vi "Gaussian surface parameter estimate.vi"(7 "output cluster":T1, 10 "X":dbl[](array[numeric]), 11 "Y":dbl[](array[numeric])) -> (3 "estimated parameters":dbl[](array[numeric]))   [LabVIEW 2023]
doc: "Estimate Gaussian surface parameters."
uses:
  <vilib>/Native 3D Graph/xcontrol/3DPC_SurfacePlot.xctl
  <vilib>/Analysis/NI_AALPro.lvlib
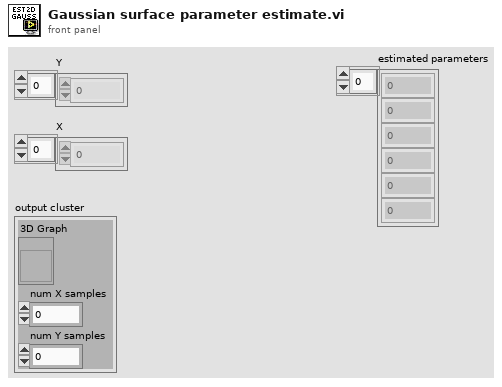
[diagram p1: front panel]
types:
  T1 = cluster{"3D Graph":refnum<vi>, "num X samples":i32, "num Y samples":i32}
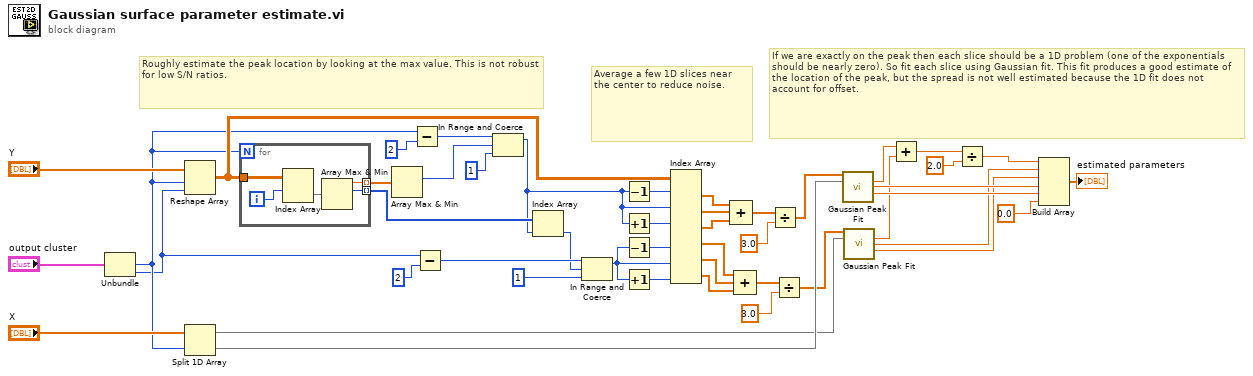
[diagram p0: block diagram]
diagram:
  # "If we are exactly on the peak then each slice should be a 1D problem (one of the exponentials should be nearly zero). So fit each slice using Gaussian fit. This fit produces a good estimate of the location of the peak, but the spread is not well estimated because the 1D fit does not account for offset."
  # "Roughly estimate the peak location by looking at the max value. This is not robust for low S/N ratios."
  # "Average a few 1D slices near the center to reduce noise."
  n1 = Unbundle("output cluster") -> ("num X samples"=w3:i32, "num Y samples"=w2:i32)  [unwired: 1 out]
  n2 = Reshape Array("Y", w3, w2) -> (w44:dbl[][])
  n3 = Split 1D Array(array="X", index=w3) -> (first subarray=w37:dbl[], second subarray=w38:dbl[])
  n4 = for {
    N: w3 -> [_]
    tunnel: w44 -> [w52]
    tunnel: [w49] -> w45 mode=indexing
    tunnel: [w48] -> w36 mode=indexing
    i -> [w51]
    n5 = Index Array(array=w52, index (row)=w51) -> (element=w50:dbl[])  [unwired: 1 in]
    n6 = Array Max & Min(array=w50) -> (max value=w49:dbl, max index (indices)=w48:i32)  [unwired: 2 out]
  }
  n7 = Array Max & Min(array=w45) -> (max index (indices)=w11:i32)  [unwired: 3 out]
  n8 = Subtract(x=w3, y=2) -> (x-y=w12:i32)
  n9 = Subtract(x=w2, y=2) -> (x-y=w7:i32)
  n10 = In Range and Coerce(upper limit=w12, x=w11, lower limit=1) -> (coerced(x)=w10:i32)  [unwired: 1 out]
  n11 = Index Array(array=w36, index=w10) -> (element=w6:i32)
  n12 = In Range and Coerce(upper limit=w7, x=w6, lower limit=1) -> (coerced(x)=w5:i32)  [unwired: 1 out]
  n13 = Decrement(x=w10) -> (x-1=w22:i32)
  n14 = Increment(x=w10) -> (x+1=w21:i32)
  n15 = Decrement(x=w5) -> (x-1=w24:i32)
  n16 = Increment(x=w5) -> (x+1=w25:i32)
  n17 = Index Array(array=w44, index (row) #1=w22, index (row) #2=w10, index (row) #3=w21, index (col) #4=w24, index (col) #5=w5, index (col) #6=w25) -> (element #1=w16:dbl[], element #2=w18:dbl[], element #3=w17:dbl[], element #4=w29:dbl[], element #5=w28:dbl[], element #6=w27:dbl[])  [unwired: 6 in]
  n18 = Compound Arithmetic op=ADD(w16, w18, w17) -> (w19:dbl[])
  n19 = Compound Arithmetic op=ADD(w29, w28, w27) -> (w30:dbl[])
  n20 = Divide(x=w19, y=3.0) -> (x/y=w15:dbl[])
  n21 = Divide(x=w30, y=3.0) -> (x/y=w23:dbl[])
  n22 = call <vilib>:"Gaussian Peak Fit.vi"("Y"=w15, "X"=w38) -> ("amplitude"=w35:dbl, "center"=w43:dbl, "standard deviation"=w42:dbl)  [unwired: 7 in, 4 out]
  n23 = call <vilib>:"Gaussian Peak Fit.vi"("Y"=w23, "X"=w37) -> ("amplitude"=w34:dbl, "center"=w41:dbl, "standard deviation"=w40:dbl)  [unwired: 7 in, 4 out]
  n24 = Add(x=w35, y=w34) -> (x+y=w33:dbl)
  n25 = Divide(x=w33, y=2.0) -> (x/y=w32:dbl)
  n26 = Build Array(w32, w41, w40, w43, w42, 0.0) -> (→"estimated parameters":dbl[])
